vi "Benchmark mupLib_eval.vi"(8 "error in (no error)":errorcluster, 10 "Iterations":i32, 11 "Expression":string) -> (0 "error out":errorcluster, 2 "x":dbl[](array[numeric]), 3 "y":dbl[](array[numeric]), 5 "dt average":dbl)   [LabVIEW 2015]
uses:
  mupLib/mupCheckError.vi
  mupLib/mupLibPath.vi
  <vilib>/Utility/error.llb/Error Cluster From Error Code.vi
  mupLib/mupLib.lvlib
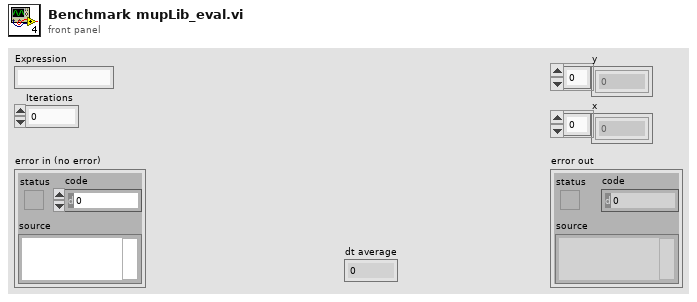
[diagram p1: front panel]
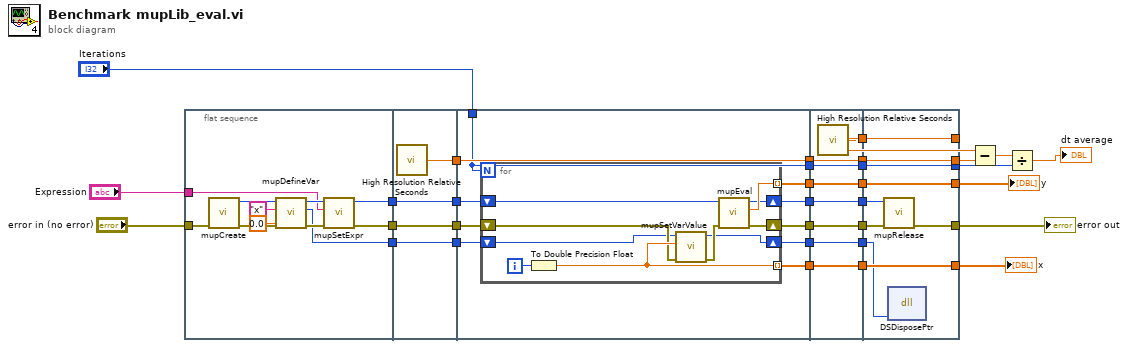
[diagram p0: block diagram]
diagram:
  n1 = flat-sequence {
    tunnel: [w35] -> w15
    tunnel: "Expression" -> [w37]
    tunnel: "error in (no error)" -> [w42]
    tunnel: [w36] -> w13
    tunnel: [w34] -> w11
    tunnel: [w48] -> w31
    tunnel: [w47] -> w26
    tunnel: w15 -> [w48]
    tunnel: [w46] -> w14
    tunnel: w13 -> [w46]
    tunnel: [w45] -> w12
    tunnel: w11 -> [w45]
    tunnel: w31 -> [w58]
    tunnel: [w57] -> w30
    tunnel: [w56] -> w29
    tunnel: [w55] -> w28
    tunnel: [w54] -> w27
    tunnel: w26 -> [w54]
    tunnel: "Iterations" -> [w53]
    tunnel: [w53] -> w20
    tunnel: w14 -> [w52]
    tunnel: w12 -> [w51]
    tunnel: [w50] -> w3
    tunnel: [w49] -> w1
    tunnel: w30 -> [w76]
    tunnel: w29 -> [w75]
    tunnel: w28 -> [w74]
    tunnel: w27 -> [w73]
    tunnel: w20 -> [w71]
    tunnel: [w76] -> w10
    tunnel: [w75] -> w9
    tunnel: [w74] -> w8
    tunnel: [w73] -> w7
    tunnel: [w72] -> w6
    tunnel: [w71] -> w5
    tunnel: [w70] -> w4
    tunnel: w3 -> [w70]
    tunnel: [w69] -> w2
    tunnel: w1 -> [w69]
    tunnel: [w81] -> w21
    tunnel: [w82] -> w25
    tunnel: [w83] -> w24
    tunnel: [w84] -> w32
    tunnel: [w85] -> w33
    tunnel: [w79] -> w16
    tunnel: w10 -> [w80]
    tunnel: w9 -> [w85]
    tunnel: w8 -> [w84]
    tunnel: w7 -> [w83]
    tunnel: w6 -> [w82]
    tunnel: w5 -> [w81]
    tunnel: w4 -> [w78]
    tunnel: w2 -> [w77]
    frame #0 {
      n2 = call "mupCreate.vi"("error in (no error)"=w42) -> ("error out"=w43:errorcluster, "hParser out"=w44:u64)  [unwired: 9 in]
      n3 = call "mupDefineVar.vi"("error in (no error)"=w43, "initValue"=0.0, "varName"="x", "hParser in"=w44) -> ("error out"=w38:errorcluster, "varAddr"=w34:u64, "hParser out"=w39:u64)  [unwired: 5 in]
      n4 = call "mupSetExpr.vi"("error in (no error)"=w38, "szExpr"=w37, "muPar in"=w39) -> ("error out"=w35:errorcluster, "muPar out"=w36:u64)  [unwired: 7 in]
    }
    frame #1 {
      n5 = call <vilib>:"High Resolution Relative Seconds.vi"() -> ("relative seconds"=w47:dbl)
    }
    frame #2 {
      n6 = for {
        N: w53 -> [_]
        shift-right: [w61] -> w57
        shift-left: w58 -> [w63]
        tunnel: [w65] -> w56 mode=indexing
        tunnel: [w66] -> w55 mode=indexing
        shift-right: [w60] -> w50
        shift-left: w52 -> [w64]
        shift-right: [w59] -> w49
        shift-left: w51 -> [w62]
        i -> [w68]
        n7 = To Double Precision Float(number=w68) -> (double precision float=w66:dbl)
        n8 = call "mupSetVarValue.vi"("error in (no error)"=w63, "varValue"=w66, "varPtr in"=w62) -> ("error out"=w67:errorcluster, "varPtr out"=w59:u64)  [unwired: 7 in]
        n9 = call "mupEval.vi"("error in (no error)"=w67, "hParser in"=w64) -> ("error out"=w61:errorcluster, "result"=w65:dbl, "hParser out"=w60:u64)  [unwired: 7 in]
      }
    }
    frame #3 {
      n10 = call <vilib>:"High Resolution Relative Seconds.vi"() -> ("relative seconds"=w72:dbl)
    }
    frame #4 {
      n11 = call "mupRelease.vi"("error in (no error)"=w80, "hParser in"=w78) -> ("error out"=w79:errorcluster)  [unwired: 9 in]
      n12 = dll-call lib="LabVIEW" fn="DSDisposePtr"("ptr"=w77) -> ()  [unwired: 5 in, 2 out]
    }
  }
  n13 = Subtract(x=w25, y=w24) -> (x-y=w22:dbl)
  n14 = Divide(x=w22, y=w21) -> (x/y=→"dt average":dbl)
  "y" <- w33
  "x" <- w32
  "error out" <- w16
